vi "Proceed Directory.vi"(8 "error in (no error)":errorcluster, 9 "path":path, 10 "Load Image Report":bool, 11 "Launch File Viewer in":refnum<class "HIJ Vision File Viewer App.lvclass">) -> (0 "error out":errorcluster, 3 "Launch File Viewer out":refnum<class "HIJ Vision File Viewer App.lvclass">)   [LabVIEW 2014, in "HIJ Vision File Viewer App.lvlib" / "HIJ Vision File Viewer App.lvclass"]
uses:
  HIJ Vision File Viewer App.lvclass
  HIJ Vision File Viewer App.lvclass/HIJ Vision File Viewer App.ctl
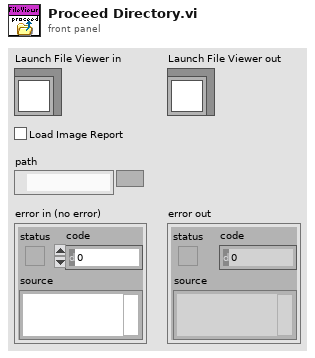
[diagram p1: front panel]
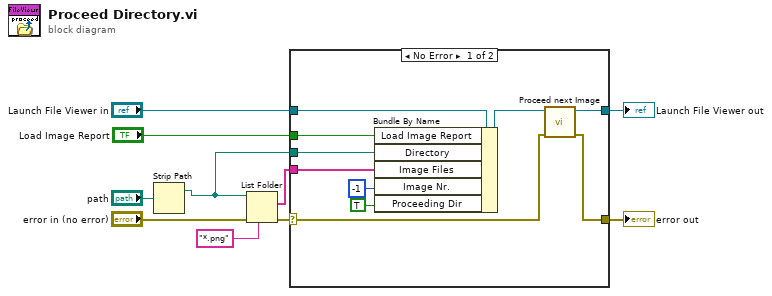
[diagram p0: block diagram]
diagram:
  n1 = Strip Path(path="path") -> (stripped path=w1:path)  [unwired: 1 out]
  n2 = List Folder(path=w1, pattern="*.png", error in="error in (no error)") -> (filenames=w5:string[], error out=w4:errorcluster)  [unwired: 1 in, 2 out]
  n3 = case shown="No Error" w4 {
    selector: w4 -> [w13 w21]
    tunnel: "Launch File Viewer in" -> [w20 w22]
    tunnel: [w14 w22] -> w8
    tunnel: w5 -> [w19 _]
    tunnel: "Load Image Report" -> [w11 _]
    tunnel: [w12 w21] -> w2
    tunnel: w1 -> [w16 _]
    frame No Error {
      n4 = Bundle By Name(cluster=w20, "Load Image Report"=w11, "Directory"=w16, "Image Files"=w19, "Image Nr."=-1, "Proceeding Dir"=TRUE) -> (w15:refnum<class "HIJ Vision File Viewer App.lvclass">)
      n5 = call-dynamic "Proceed next Image.vi"("error in (no error)"=w13, "Launch File Viewer in"=w15) -> ("error out"=w12:errorcluster, "Launch File Viewer out"=w14:refnum<class "HIJ Vision File Viewer App.lvclass">)  [unwired: 8 in]
    }
    frame Error {
    }
  }
  "error out" <- w2
  "Launch File Viewer out" <- w8
